vi "Select_operator.vi"(0 "Enable":bool=TRUE, 1 "sub vi?":bool, 5 "error in (no error)":errorcluster, 6 "small?":bool) -> (14 "Operator Cluster 2":T1 {"Operator" items=["Giraffe", "Andrew Collette", "Keith Drake", "Anthony Shu", "Evan Thomas", "Nicholaus Beaty", "David James", "John Fontanese", ""]}, 18 "OK":bool, 19 "error out":errorcluster)   [LabVIEW 2013]
doc: "Displays a standard dialog box that prompts users to enter information, such as a user name and password.\n--------------------\n\nThis Express VI is configured as follows:\n\nMessage to Display to the User:Select Operator:\nThe inputs are:"
uses:
  Controls/Operator.ctl
  <vilib>/addons/database/Auxilliary.llb/DB Tools Cursor Type.ctl
  <vilib>/Utility/miscctls.llb/LVPointTypeDef.ctl
  <vilib>/addons/database/Connection.llb/Conn Execute.vi
  <vilib>/addons/database/Recordset.llb/Rec Fetch Recordset Data (R).vi
  <vilib>/addons/database/Recordset.llb/Rec Destroy - Connection.vi
  <vilib>/addons/database/_DB Variant To Data/Database Variant To Data.xnode
  <vilib>/addons/database/NI_Database_API.lvlib
panel:
  in  "Operator Cluster":T1 {"Operator" items=["Giraffe", "Andrew Collette", "Keith Drake", "Anthony Shu", "Evan Thomas", "Nicholaus Beaty", "David James", "John Fontanese", ""]}
  out "String":string="Select Operator:"
  in  "Cancel":bool
  in  "OK2":bool
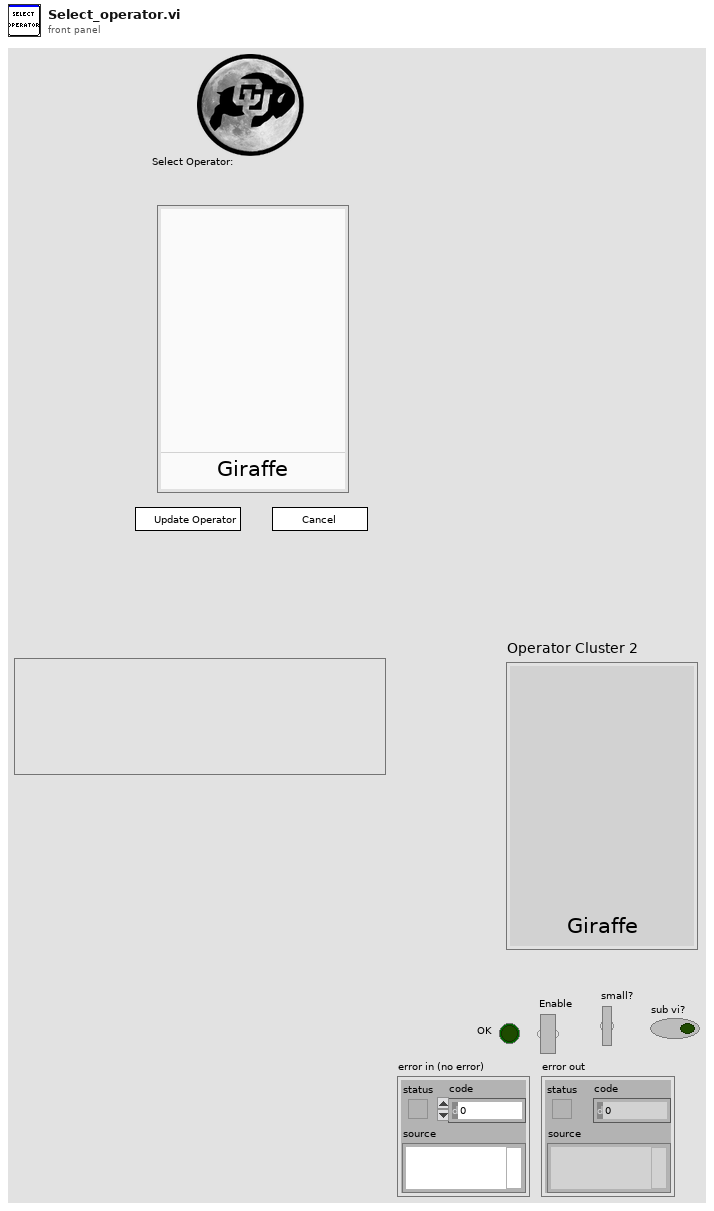
[diagram p1: front panel]
types:
  T1 = typedef "Operator.ctl" = cluster{"Timestamp":i64, "Operator":u16}
  T2 = typedef "LVPointTypeDef.ctl" = cluster{"Horizontal":i16, "Vertical":i16}
  T3 = typedef "NI_Database_API.lvlib/DB Tools Cursor Type.ctl" = enum16{"forward-only", "keyset", "dynamic", "static"}
  T4 = cluster{"Input Name":string, "Input Data Type":i32}[]
  T5 = typedef "NI_Database_API.lvlib/Conn ObjectReference.ctl" = refnum<k1>
  T6 = typedef "NI_Database_API.lvlib/Rec ObjectReference.ctl" = refnum<k1>
  T7 = enum32{"Invalid", "Standard", "Closed", "Hidden", "Minimized", "Maximized"}
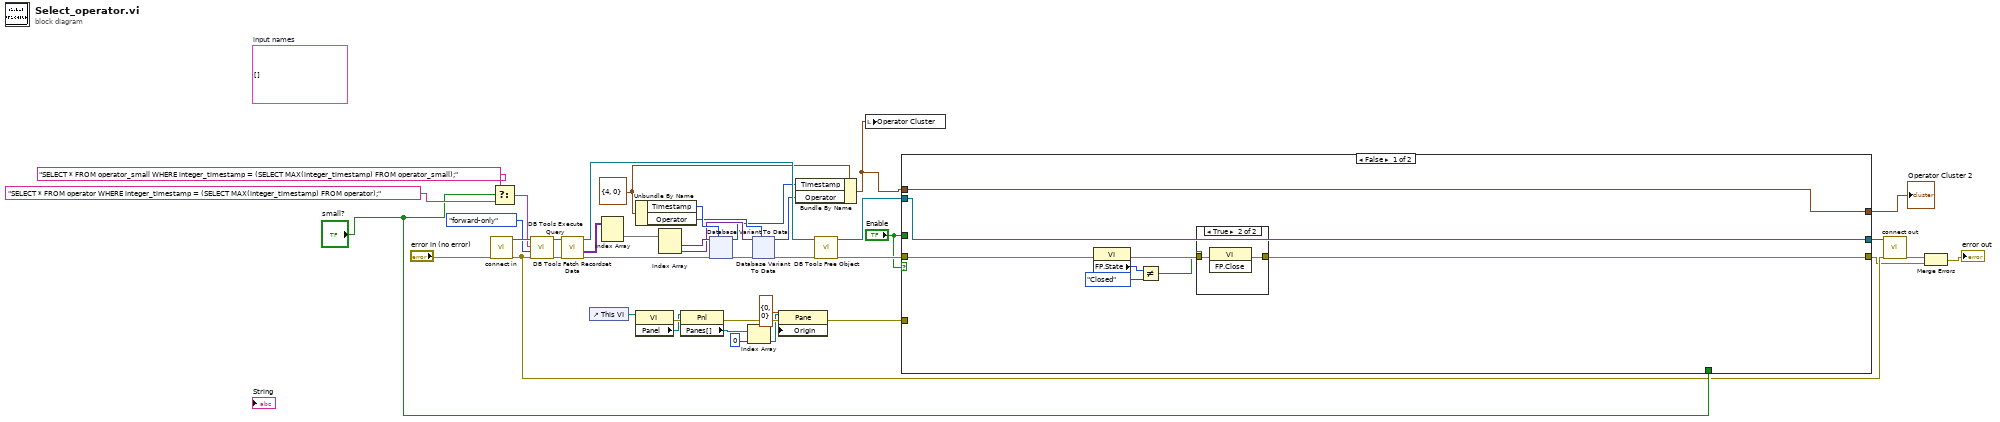
[diagram p0: block diagram]
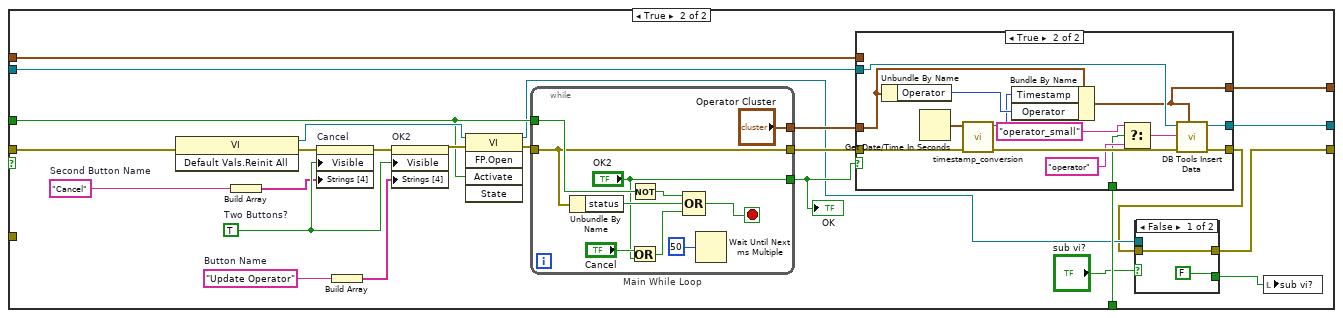
[diagram p3: hidden frame]
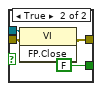
[diagram p4: hidden frame]
diagram:
  w20 = T1 {"Timestamp"=4, "Operator"=0} ("Operator Cluster")
  (unwired) T4 []  # input names
  n1 = call "connect in.vi"("error in (no error)"="error in (no error)") -> ("error out"=w12:errorcluster, "Database Connection"=w37:T5)  [unwired: 6 in, 1 out]
  n2 = Select(t="SELECT * FROM operator_small WHERE integer_timestamp = (SELECT MAX(integer_timestamp) FROM operator_small);" ("table"), s="small?", f="SELECT * FROM operator WHERE integer_timestamp = (SELECT MAX(integer_timestamp) FROM operator);" ("table")) -> (s? t:f=w14:string)
  n3 = call-poly <vilib>:"DB Tools Execute Query.vi"("error in (no error)"=w12, "cursor type"=DB_Tools_Cursor_Type."forward-only", "SQL query"=w14, "connection reference"=w37) -> ("error out"=w38:errorcluster, "recordset reference"=w36:T6)  [unwired: 4 in]
  n4 = call-poly <vilib>:"DB Tools Fetch Recordset Data.vi"("error in (no error)"=w38, "recordset reference"=w36) -> ("error out"=w27:errorcluster, "recordset data"=w33:variant[][], "recordset reference out"=w25:T6)  [unwired: 3 in]
  n5 = control-ref of="This VI"() -> (w9:refnum<vi>)
  n6 = Index Array(array=w33) -> (element=w30:variant[])  [unwired: 2 in]
  n7 = Unbundle By Name(w20) -> ("Timestamp"=w32:i64, "Operator"=w31:u16)
  n8 = property class="VI"(reference=w9) -> (error out=w8:errorcluster, "Panel"=w7:refnum<vi>)  [unwired: 1 in, 1 out]
  n9 = Index Array(array=w30) -> (element #1=w29:variant, element #2=w28:variant)  [unwired: 2 in]
  n10 = property class="Pnl"(reference=w7, error in=w8) -> (error out=w6:errorcluster, "Panes[]"=w5:refnum<vi>[])  [unwired: 1 out]
  n11 = xnode "Database Variant To Data"("database variant"=w29, "error in (no error)"=w27, "type"=w32) -> ("data"=w24:i64, "error out"=w34:errorcluster)
  n12 = Index Array(array=w5, index=0) -> (element=w3:refnum<vi>)
  n13 = xnode "Database Variant To Data"("database variant"=w28, "error in (no error)"=w34, "type"=w31) -> ("data"=w23:u16, "error out"=w26:errorcluster)
  n14 = property class="Pane"(reference=w3, error in=w6, "Origin"=T2 {"Horizontal"=0, "Vertical"=0}) -> (error out=w1:errorcluster)  [unwired: 1 out]
  n15 = Bundle By Name(cluster=w20, "Timestamp"=w24, "Operator"=w23) -> (w18:T1)
  n16 = call-poly <vilib>:"DB Tools Free Object.vi"("error in (no error)"=w26, "recordset reference"=w25) -> ("error out"=w22:errorcluster, "connection reference"=w21:T5)  [unwired: 8 in]
  n17 = local write "Operator Cluster"(w18) -> ()
  n18 = case shown="False" "Enable" {
    tunnel: [w49 w68] -> w41
    tunnel: [w47 w55] -> w10
    tunnel: [w48 w67] -> w39
    tunnel: w18 -> [w49 w66]
    tunnel: w22 -> [w46 w65]
    tunnel: w21 -> [w48 w63]
    tunnel: "Enable" -> [_ w58]
    tunnel: "small?" -> [_ w62]
    tunnel: w1 -> [_ _]
    frame False {
      n19 = property class="VI"(error in=w46) -> (error out=w45:errorcluster, "FP.State"=w44:T7)  [unwired: 1 in, 1 out]
      n20 = Not Equal?(x=w44, y=T7."Closed") -> (x != y?=w42:bool)
      n21 = case shown="True" w42 {
        tunnel: [w50 w52] -> w47
        tunnel: w45 -> [w50 w51]
        frame False {
        }
        frame True {
          n22 = invoke class="VI" method="FP.Close"(error in=w51) -> (error out=w52:errorcluster)  [unwired: 2 in, 2 out]
        }
      }
    }
    frame True {
      w74 = "Cancel"  # Second Button Name
      w72 = "Update Operator"  # Button Name
      w77 = TRUE  # Two Buttons?
      n23 = invoke class="VI" method="Default Vals.Reinit All"(error in=w65) -> (reference out=w61:refnum<vi>, error out=w64:errorcluster)  [unwired: 2 in, 1 out]
      n24 = Build Array(w74) -> (w75:string[])
      n25 = property on="Cancel" class="Bool"(error in=w64, "Visible"=w77, "Strings [4]"=w75) -> (error out=w76:errorcluster)  [unwired: 1 in, 1 out]
      n26 = Build Array(w72) -> (w73:string[])
      n27 = property on="OK2" class="Bool"(error in=w76, "Visible"=w77, "Strings [4]"=w73) -> (error out=w60:errorcluster)  [unwired: 1 in, 1 out]
      n28 = invoke class="VI" method="FP.Open"(reference=w61, error in=w60, "Activate"=w58) -> (reference out=w57:refnum<vi>, error out=w59:errorcluster)  [unwired: 2 in, 3 out]
      n29 = while "Main While Loop" {
        tunnel: ["OK2"] -> w70
        tunnel: w58 -> [w108]
        tunnel: w59 -> [w105]
        tunnel: [w105] -> w71
        tunnel: ["Operator Cluster"] -> w69
        stop <- w106 stop-if-true
        n30 = Unbundle By Name(w105) -> ("status"=w103:bool)
        n31 = Not(x=w108) -> (.not. x?=w107:bool)
        n32 = Or(x="Cancel", y="OK2") -> (x .or. y?=w104:bool)
        n33 = Compound Arithmetic op=OR(w107, w103, w104) -> (w106:bool)
        n34 = Wait Until Next ms Multiple(millisecond multiple=u32 50) -> ()  [unwired: 1 out]
      }
      "OK" <- w70
      n35 = case shown="True" w70 {
        tunnel: w71 -> [w86 w98]
        tunnel: [w86 w95] -> w56
        tunnel: w69 -> [_ w91]
        tunnel: [w85 w94] -> w68
        tunnel: w63 -> [w84 w96]
        tunnel: w66 -> [w85 _]
        tunnel: [w84 w93] -> w67
        tunnel: w62 -> [_ w88]
        frame False {
        }
        frame True {
          n36 = Unbundle By Name(w91) -> ("Operator"=w100:u16)
          n37 = Get Date/Time In Seconds() -> (seconds since 1Jan1904=w99:timestamp)
          n38 = call "timestamp_conversion.vi"("error in (no error)"=w98, "Time Stamp"=w99) -> ("error out"=w97:errorcluster, "Integer Time"=w92:i64)  [unwired: 7 in]
          n39 = Bundle By Name(cluster=w91, "Timestamp"=w92, "Operator"=w100) -> (w94:T1)
          n40 = Select(t="operator_small" ("table"), s=w88, f="operator" ("table")) -> (s? t:f=w87:string)
          n41 = call <vilib>:"DB Tools Insert Data.vi"("data"=w94, "error in (no error)"=w97, "table"=w87, "connection reference"=w96) -> ("error out"=w95:errorcluster, "connection reference out"=w93:T5)  [unwired: 6 in]
        }
      }
      n42 = case shown="False" "sub vi?" {
        tunnel: w57 -> [_ w83]
        tunnel: w56 -> [w79 w82]
        tunnel: [w79 w81] -> w55
        tunnel: [FALSE ("sub vi?") FALSE ("sub vi?")] -> w53
        frame False {
        }
        frame True {
          n43 = invoke class="VI" method="FP.Close"(reference=w83, error in=w82) -> (error out=w81:errorcluster)  [unwired: 1 in, 2 out]
        }
      }
      n44 = local write "sub vi?"(w53) -> ()
    }
  }
  "Operator Cluster 2" <- w41
  n45 = call "connect out.vi"("error in (no error)"=w12, "connection reference"=w39) -> ("error out"=w17:errorcluster)  [unwired: 9 in]
  n46 = Merge Errors(w17, w10) -> (→"error out":errorcluster)
